vi "Test1.vi"() -> ()   [LabVIEW 2016, in "Data Saving.lvlib" / "Data Saver.lvclass"]
uses:
  TDMS Saver/Data Saver.lvclass
  C:/Program Files (x86)/National Instruments/LabVIEW 2016/vi.lib/ActorFramework/Actor/Actor.lvclass
  <vilib>/ActorFramework/Message Enqueuer/Message Enqueuer.lvclass/Message Enqueuer.ctl
  Data Saver Messages/Write data to Signal Ref Msg/Write data to Signal Ref Msg.lvclass/Write data to Signal Ref Msg.ctl
  <vilib>/ActorFramework/Message Enqueuer/Enqueue.vi
  <vilib>/ActorFramework/Stop Msg/Stop Msg.lvclass
  C:/Program Files (x86)/National Instruments/LabVIEW 2016/vi.lib/ActorFramework/Message/Message.lvclass
  Data Saver Messages/Write data to Signal Ref Msg/Write data to Signal Ref Msg.lvclass
  <vilib>/ActorFramework/Message Priority Queue/Priority Enqueue.vi
  <vilib>/ActorFramework/Actor/Actor.lvclass
panel:
  in  "Record Button":bool
  in  "Stop Button":bool
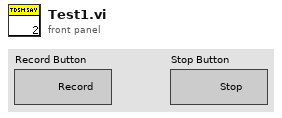
[diagram p1: front panel]
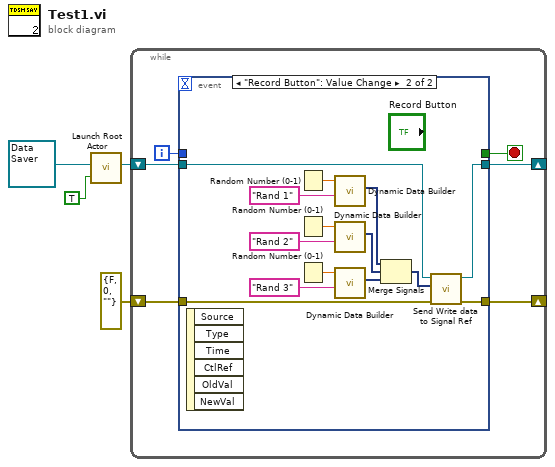
[diagram p0: block diagram]
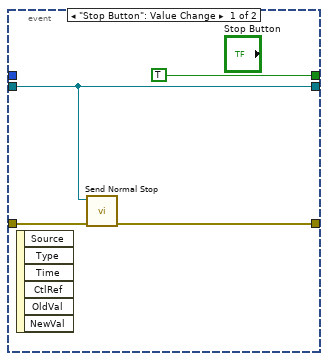
[diagram p2: hidden frame]
diagram:
  n1 = call <vilib>:"Launch Root Actor.vi"("Open Actor Core front panel? (F)"=TRUE, "Actor"=refnum<class "Data Saver.lvclass"> refnum ("Data Saving.lvlib:Data Saver.lvclass")) -> ("Actor's Enqueuer"=w2:refnum<class "Message Enqueuer.lvclass">)  [unwired: 8 in, 1 out]
  n2 = while {
    shift-right: [w8] -> _
    shift-left: w2 -> [w10]
    shift-right: [w7] -> _
    shift-left: errorcluster {"status"=FALSE, "code"=0, "source"=""} ("error out") -> [w6]
    i -> [w5]
    stop <- w9 stop-if-true
    n3 = event shown="[1] \"Record Button\": Value Change" {
      selector: _ -> [_ _]
      dyn-events: _ -> [_ _]
      timeout: _ -> [_ _]
      tunnel: w10 -> [w13 w28]
      tunnel: [TRUE _] -> w9
      tunnel: [w13 w25] -> w8
      tunnel: [w12 w26] -> w7
      tunnel: w6 -> [w11 w27]
      tunnel: w5 -> [_ _]
      event "Stop Button": Value Change {
        n4 = event-data() -> ()  [unwired: 1 in, 6 out]
        n5 = call <vilib>:"Send Normal Stop.vi"("error in (no error)"=w11, "Message Enqueuer"=w13) -> ("error out"=w12:errorcluster)  [unwired: 9 in]
      }
      event "Record Button": Value Change {
        n6 = event-data() -> ()  [unwired: 1 in, 6 out]
        n7 = Random Number (0-1)() -> (number: 0 to 1=w24:dbl)
        n8 = Random Number (0-1)() -> (number: 0 to 1=w21:dbl)
        n9 = Random Number (0-1)() -> (number: 0 to 1=w17:dbl)
        n10 = call "Dynamic Data Builder.vi"("Signal Name"="Rand 1", "Number in"=w24) -> ("Dynamic Signame Out"=w20:dynamicdata)  [unwired: 9 in]
        n11 = call "Dynamic Data Builder.vi"("Signal Name"="Rand 2", "Number in"=w21) -> ("Dynamic Signame Out"=w19:dynamicdata)  [unwired: 9 in]
        n12 = call "Dynamic Data Builder.vi"("Signal Name"="Rand 3", "Number in"=w17) -> ("Dynamic Signame Out"=w15:dynamicdata)  [unwired: 9 in]
        n13 = Merge Signals(w20, w19, w15) -> (w18:dynamicdata)
        n14 = call "Send Write data to Signal Ref.vi"("error in (no error)"=w27, "Waveform Graph"=w18, "Message Enqueuer"=w28) -> ("error out"=w26:errorcluster, "Message Enqueuer out"=w25:refnum<class "Message Enqueuer.lvclass">)  [unwired: 7 in]
      }
    }
  }
